vi "tab control refresh.vi"(8 "error in":errorcluster, 9 "write directory":path, 10 "read directory":path, 11 "VI reference":refnum<vi>) -> (0 "error out":errorcluster)   [LabVIEW 2013, in "Shared Memory Editor Node.lvclass"]
doc: "Copyright 2016 National Instruments Corporation\n\nLicensed under the Apache License, Version 2.0 (the \"License\"); you may not use this file except in compliance with the License. You may obtain a copy of the License at http://www.apache.org/licenses/LICENSE-2.0\nUnless required by applicable law or agreed to in writing, software distributed under the License is distributed on an \"AS IS\" BASIS, WITHOUT WARRANTIES OR CONDITIONS OF ANY KIND, either express or implied. See the License for the specific language governing permissions and limitations under the License."
uses:
  Shared Memory Editor Node.lvclass
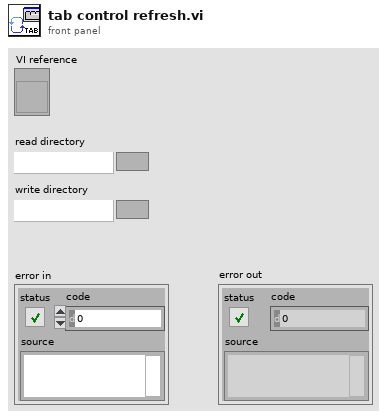
[diagram p1: front panel]
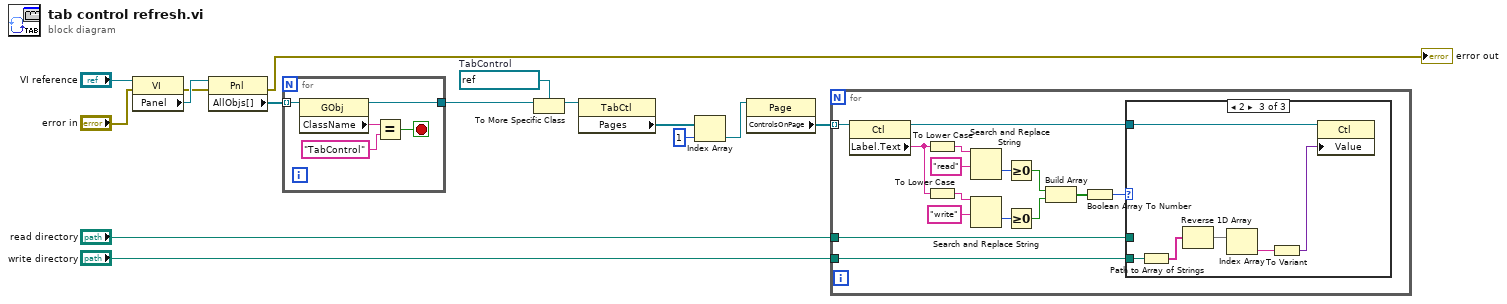
[diagram p0: block diagram]
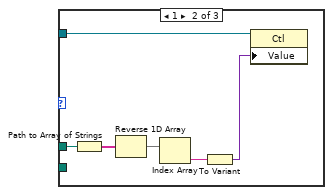
[diagram p3: hidden frame]
diagram:
  w10 = refnum<vi> refnum  # TabControl
  n1 = property class="VI"(reference="VI reference", error in="error in") -> (error out=w6:errorcluster, "Panel"=w8:refnum<vi>)  [unwired: 1 out]
  n2 = property class="Pnl"(reference=w8, error in=w6) -> (error out=→"error out":errorcluster, "AllObjs[]"=w7:refnum<vi>[])  [unwired: 1 out]
  n3 = for {
    tunnel: w7 -> [w20] mode=indexing
    tunnel: [w19] -> w9
    stop <- w16 stop-if-true
    n4 = property class="GObj"(reference=w20) -> (reference out=w19:refnum<vi>, "ClassName"=w17:string)  [unwired: 1 in, 1 out]
    n5 = Equal?(x=w17, y="TabControl") -> (x = y?=w16:bool)
  }
  n6 = To More Specific Class(target class=w10, reference=w9) -> (specific class reference=w11:refnum<vi>)  [unwired: 1 in, 1 out]
  n7 = property class="TabCtl"(reference=w11) -> ("Pages"=w12:refnum<vi>[])  [unwired: 1 in, 2 out]
  n8 = Index Array(array=w12, index=1) -> (element=w14:refnum<vi>)
  n9 = property class="Page"(reference=w14) -> ("ControlsOnPage"=w15:refnum<vi>[])  [unwired: 1 in, 2 out]
  n10 = for {
    tunnel: w15 -> [w35] mode=indexing
    tunnel: "read directory" -> [w22]
    tunnel: "write directory" -> [w21]
    n11 = property class="Ctl"(reference=w35) -> (reference out=w34:refnum<vi>, "Label.Text"=w29:string)  [unwired: 1 in, 1 out]
    n12 = To Lower Case(string=w29) -> (all lower case string=w33:string)
    n13 = To Lower Case(string=w29) -> (all lower case string=w30:string)
    n14 = Search and Replace String(input string=w33, search string="read") -> (offset past replacement=w28:i32)  [unwired: 6 in, 3 out]
    n15 = Search and Replace String(input string=w30, search string="write") -> (offset past replacement=w27:i32)  [unwired: 6 in, 3 out]
    n16 = Greater Or Equal To 0?(x=w28) -> (x >= 0?=w26:bool)
    n17 = Greater Or Equal To 0?(x=w27) -> (x >= 0?=w25:bool)
    n18 = Build Array(w26, w25) -> (w24:bool[])
    n19 = Boolean Array To Number(Boolean array=w24) -> (number=w23:u32)
    n20 = case shown="2" w23 {
      tunnel: w34 -> [_ w41 w47]
      tunnel: w22 -> [_ w39 _]
      tunnel: w21 -> [_ _ w42]
      frame Default {
      }
      frame 1 {
        n21 = Path to Array of Strings(0:w39) -> (2:w38:string[])  [unwired: 1 out]
        n22 = Reverse 1D Array(array=w38) -> (reversed array=w37:string[])
        n23 = Index Array(array=w37) -> (element=w36:string)  [unwired: 1 in]
        n24 = To Variant(anything=w36) -> (Variant=w40:variant)
        n25 = property class="Ctl"(reference=w41, "Value"=w40) -> ()  [unwired: 1 in, 2 out]
      }
      frame 2 {
        n26 = Path to Array of Strings(0:w42) -> (2:w45:string[])  [unwired: 1 out]
        n27 = Reverse 1D Array(array=w45) -> (reversed array=w44:string[])
        n28 = Index Array(array=w44) -> (element=w43:string)  [unwired: 1 in]
        n29 = To Variant(anything=w43) -> (Variant=w46:variant)
        n30 = property class="Ctl"(reference=w47, "Value"=w46) -> ()  [unwired: 1 in, 2 out]
      }
    }
  }
